vi "Agilent VNA Set Trace Display.vi"(4 "Trace":i8=1 min=1 max=99 step=1, 6 "Channel":i8=1 min=1 max=99 step=1, 7 "Agilent VNA":T1, 8 "error in (no error)":errorcluster, 11 "VISA Resource Name":refnum<visa-resource-name>) -> (0 "error out":errorcluster, 2 "Measurements":string[](array[string]), 3 "dup VISA Resource Name":refnum<visa-resource-name>)   [LabVIEW 2011]
uses:
  TypeDefs/Agilent VNA Instrument Info.ctl
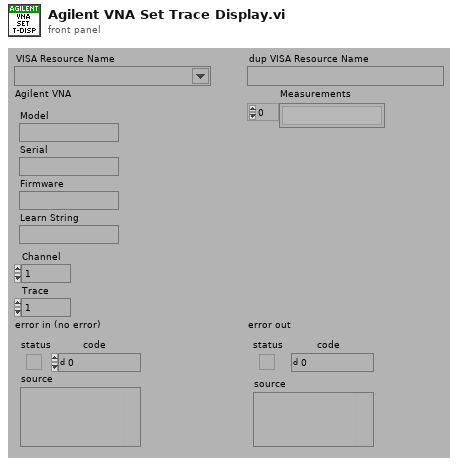
[diagram p1: front panel]
types:
  T1 = typedef "Agilent VNA Instrument Info.ctl" = cluster{"Model":string, "Serial":string, "Firmware":string, "Learn String":string}
  T2 = typedef "Agilent VNA Model.ctl" = enum16{"Not Supported", "8510X", "8719X", "8720X", "8722X", "8753X", "ENA", "PNA", "Field Fox"}
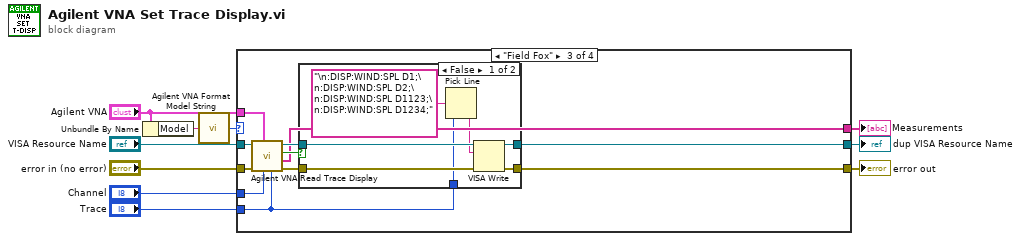
[diagram p0: block diagram]
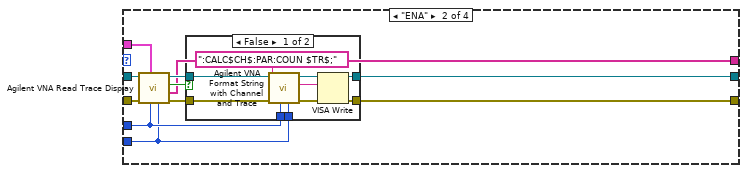
[diagram p3: hidden frame]
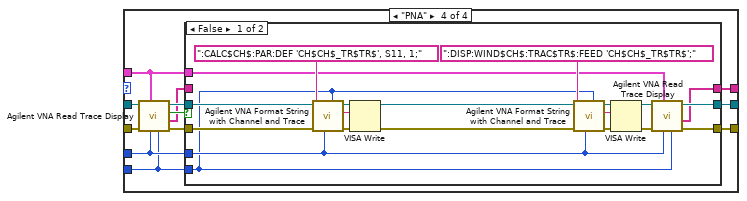
[diagram p6: hidden frame]
diagram:
  n1 = Unbundle By Name("Agilent VNA") -> ("Model"=w3:string)
  n2 = call "Agilent VNA Format Model String.vi"("Model"=w3) -> ("Model"=w6:T2)
  n3 = case shown="\"Field Fox\"" w6 {
    tunnel: "VISA Resource Name" -> [w12 w20 w41 w62]
    tunnel: "error in (no error)" -> [w11 w21 w42 w63]
    tunnel: [w12 w23 w44 w65] -> w8
    tunnel: [w11 w22 w43 w64] -> w7
    tunnel: "Channel" -> [_ w16 w37 w59]
    tunnel: "Agilent VNA" -> [_ w17 w38 w55]
    tunnel: "Trace" -> [_ w15 w36 w58]
    tunnel: [_ w13 w34 w54] -> w1
    frame "Not Supported".."8753X" {
    }
    frame "ENA" {
      n4 = call "Agilent VNA Read Trace Display.vi"("Trace"=w15, "Channel"=w16, "Agilent VNA"=w17, "error in (no error)"=w21, "VISA Resource Name"=w20) -> ("error out"=w18:errorcluster, "Measurements"=w13:string[], "Displayed?"=w14:bool, "dup VISA Resource Name"=w19:refnum<visa-resource-name>)  [unwired: 3 out]
      n5 = case shown="False" w14 {
        tunnel: [w31 w33] -> w23
        tunnel: [w30 w32] -> w22
        tunnel: w19 -> [w29 w33]
        tunnel: w18 -> [w28 w32]
        tunnel: w16 -> [w26 _]
        tunnel: w15 -> [w25 _]
        frame False {
          n6 = call "Agilent VNA Format String with Channel and Trace.vi"("Trace"=w25, "Channel"=w26, "String"=":CALC$CH$:PAR:COUN $TR$;" ("write buffer")) -> ("String Out"=w27:string)  [unwired: 6 out]
          n7 = VISA Write(VISA resource name=w29, write buffer=w27, error in (no error)=w28) -> (VISA resource name out=w31:refnum<visa-resource-name>, error out=w30:errorcluster)  [unwired: 1 out]
        }
        frame True {
        }
      }
    }
    frame "Field Fox" {
      n8 = call "Agilent VNA Read Trace Display.vi"("Trace"=w36, "Channel"=w37, "Agilent VNA"=w38, "error in (no error)"=w42, "VISA Resource Name"=w41) -> ("error out"=w39:errorcluster, "Measurements"=w34:string[], "Displayed?"=w35:bool, "dup VISA Resource Name"=w40:refnum<visa-resource-name>)  [unwired: 3 out]
      n9 = case shown="False" w35 {
        tunnel: [w51 w53] -> w44
        tunnel: [w50 w52] -> w43
        tunnel: w40 -> [w49 w53]
        tunnel: w39 -> [w48 w52]
        tunnel: w36 -> [w45 _]
        frame False {
          n10 = Pick Line(multi-line string="\n:DISP:WIND:SPL D1;\n:DISP:WIND:SPL D2;\n:DISP:WIND:SPL D1123;\n:DISP:WIND:SPL D1234;" ("write buffer"), line index=w45) -> (output string=w46:string)  [unwired: 1 in]
          n11 = VISA Write(VISA resource name=w49, write buffer=w46, error in (no error)=w48) -> (VISA resource name out=w51:refnum<visa-resource-name>, error out=w50:errorcluster)  [unwired: 1 out]
        }
        frame True {
        }
      }
    }
    frame "PNA" {
      n12 = call "Agilent VNA Read Trace Display.vi"("Trace"=w58, "Channel"=w59, "Agilent VNA"=w55, "error in (no error)"=w63, "VISA Resource Name"=w62) -> ("error out"=w60:errorcluster, "Measurements"=w56:string[], "Displayed?"=w57:bool, "dup VISA Resource Name"=w61:refnum<visa-resource-name>)  [unwired: 3 out]
      n13 = case shown="False" w57 {
        tunnel: [w71 w84] -> w65
        tunnel: [w72 w83] -> w64
        tunnel: w61 -> [w80 w84]
        tunnel: w60 -> [w81 w83]
        tunnel: w59 -> [w68 _]
        tunnel: w58 -> [w67 _]
        tunnel: w56 -> [_ w82]
        tunnel: w55 -> [w69 _]
        tunnel: [w66 w82] -> w54
        frame False {
          n14 = call "Agilent VNA Format String with Channel and Trace.vi"("Trace"=w67, "Channel"=w68, "String"=":CALC$CH$:PAR:DEF 'CH$CH$_TR$TR$', S11, 1;" ("write buffer")) -> ("String Out"=w79:string)  [unwired: 6 out]
          n15 = VISA Write(VISA resource name=w80, write buffer=w79, error in (no error)=w81) -> (VISA resource name out=w77:refnum<visa-resource-name>, error out=w76:errorcluster)  [unwired: 1 out]
          n16 = call "Agilent VNA Format String with Channel and Trace.vi"("Trace"=w67, "Channel"=w68, "String"=":DISP:WIND$CH$:TRAC$TR$:FEED 'CH$CH$_TR$TR$';" ("write buffer")) -> ("String Out"=w78:string)  [unwired: 6 out]
          n17 = VISA Write(VISA resource name=w77, write buffer=w78, error in (no error)=w76) -> (VISA resource name out=w70:refnum<visa-resource-name>, error out=w73:errorcluster)  [unwired: 1 out]
          n18 = call "Agilent VNA Read Trace Display.vi"("Trace"=w67, "Channel"=w68, "Agilent VNA"=w69, "error in (no error)"=w73, "VISA Resource Name"=w70) -> ("error out"=w72:errorcluster, "Measurements"=w66:string[], "dup VISA Resource Name"=w71:refnum<visa-resource-name>)  [unwired: 4 out]
        }
        frame True {
        }
      }
    }
  }
  "dup VISA Resource Name" <- w8
  "error out" <- w7
  "Measurements" <- w1
